vi "tvac_gui.vi"() -> ()   [LabVIEW 2017]
uses:
  <vilib>/httpClient/ClientHandle.ctl
  msg7171_linux.llb/send single message.vi
  <vilib>/httpClient/POSTBuffer.vi
  <vilib>/httpClient/LabVIEWHTTPClient.lvlib
panel:
  out "Index Values":u32[](array[numeric])
  in  "Subtractor":i32=10
  in  "index (col)":i32
  in  "alarm":i32
  in  "NumberTCs":i32=120
  in  "Tab Control":enum32{"Page 1", "Page 2"}(tab)
  in  "Zone 1":T1 {"Ring" items=["Average", "Maximum", "Minimum", ""]}
  in  "Graphing Selection":u16(ring) items=["User Selection", "Graph All Thermocouples", "Clear Graph"]
  in  "Time Scale":u16(ring) items=["Minutes", "Hours", "Seconds"]
  out "Waveform Chart":waveform(dbl)[](graph)
  out "Thermocouples":T2(array[cluster])
  in  "exit":bool
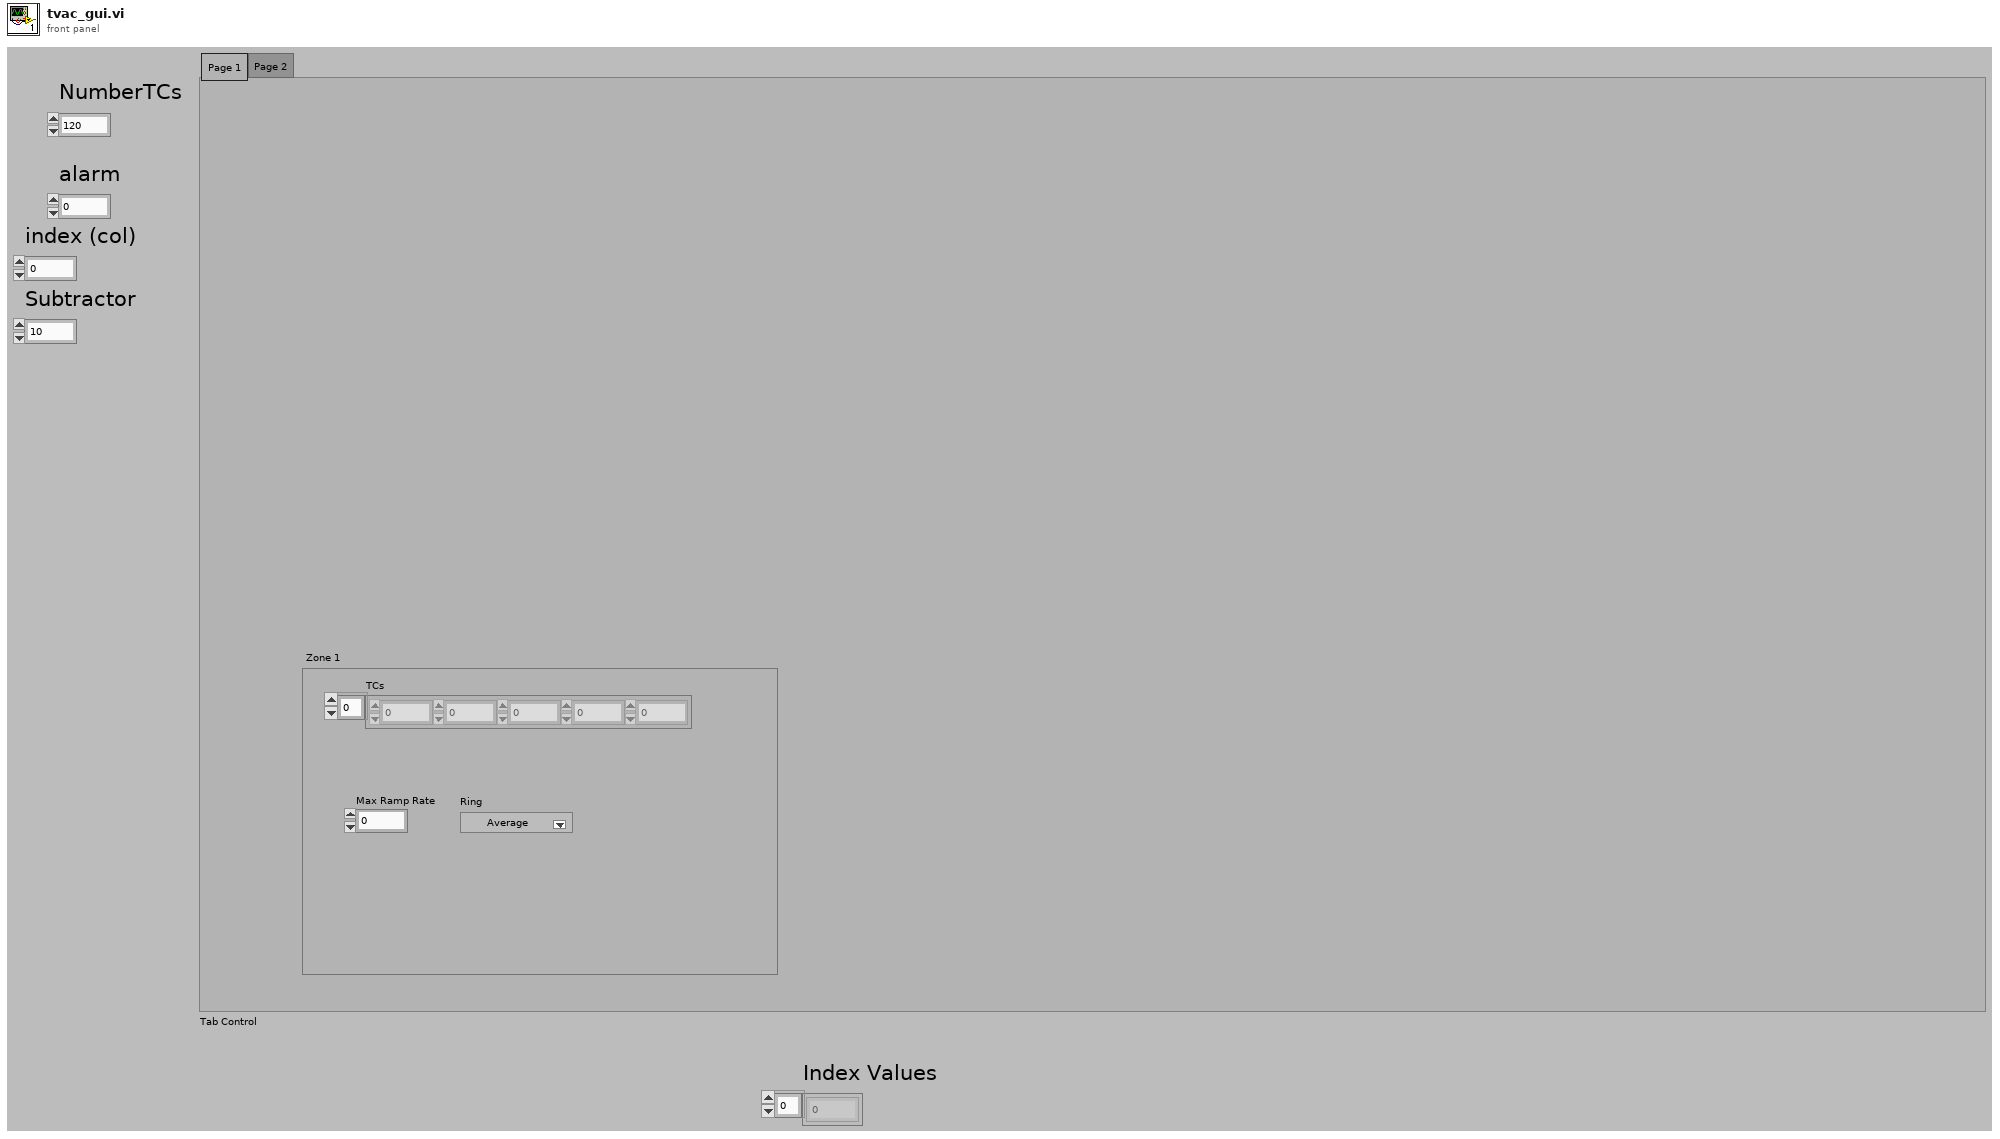
[diagram p1: front panel]
types:
  T1 = cluster{"Ring":u16, "Max Ramp Rate":dbl, "TCs":dbl[]}
  T2 = cluster{"TC Label":string, "Alarm Status":string, "Alarm Color":u32, "Temperature":string, "PlotColor":u32, "Graph On/Off":u32}[][]
  T3 = typedef "LabVIEWHTTPClient.lvlib/ClientHandle.ctl" = refnum<k1>
  T4 = cluster{"go":bool, "Http session":T3, "URL prefex":string}
  T5 = typedef "LVPoint32TypeDef.ctl" = cluster{"Horizontal":i32, "Vertical":i32}
  T6 = typedef "LVPositionTypeDef.ctl" = cluster{"Left":i32, "Top":i32}
  T7 = cluster{"TC Label":string, "Alarm Status":string, "Alarm Color":u32, "Temperature":string, "PlotColor":u32, "Graph On/Off":u32}
  T8 = typedef "LVRangeTypeDef.ctl" = cluster{"Minimum":dbl, "Maximum":dbl, "Increment":dbl, "Minor Increment":dbl, "Start":dbl}
  T9 = cluster{"time":string, "tcs":cluster{"thermocouple":i32, "time":i32, "temp":i32, "working":bool, "alarm":i32}[]}
  T10 = cluster{"thermocouple":i32, "time":i32, "temp":i32, "working":bool, "alarm":i32}[]
  T11 = cluster{"thermocouple":i32, "time":i32, "temp":i32, "working":bool, "alarm":i32}
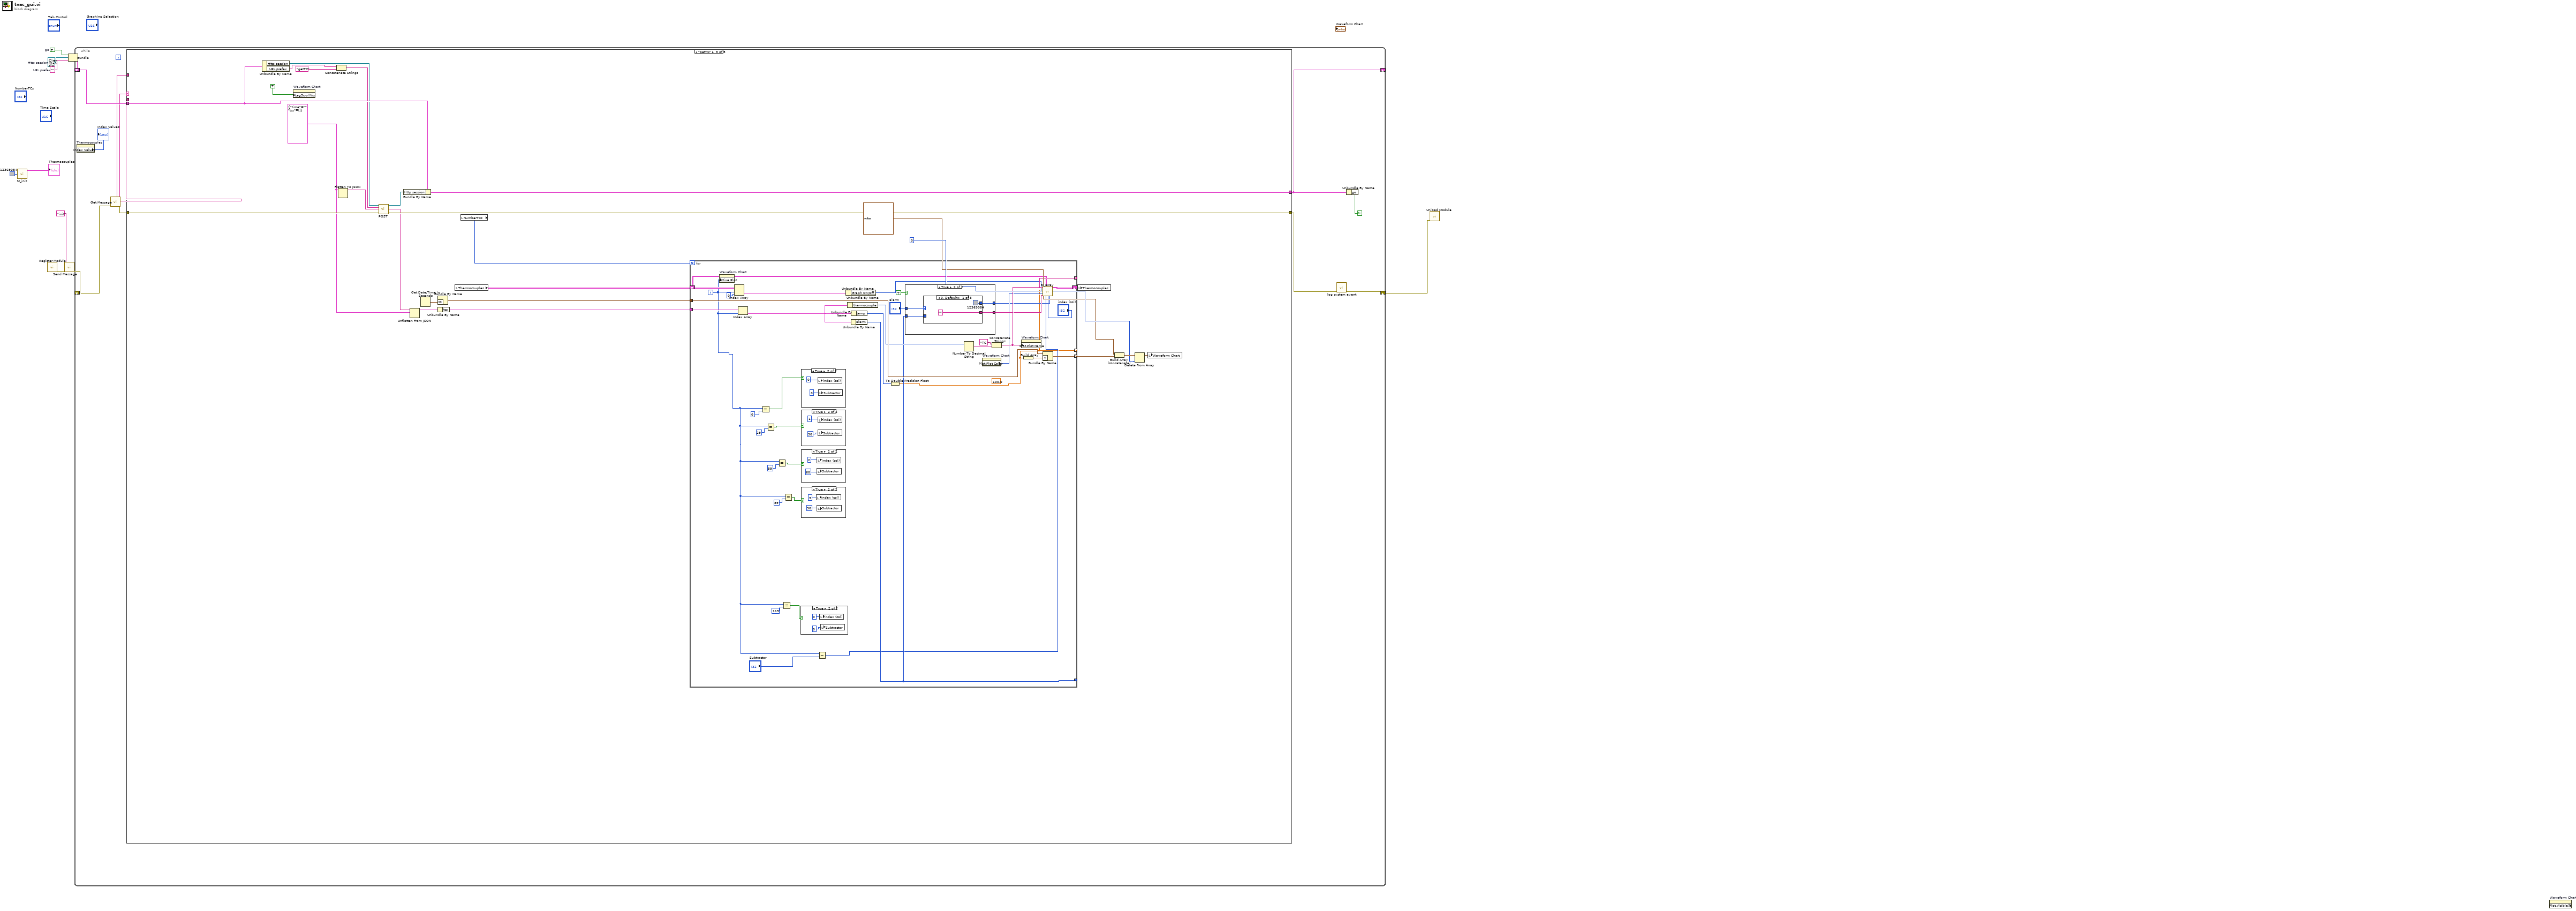
[diagram p0: block diagram]
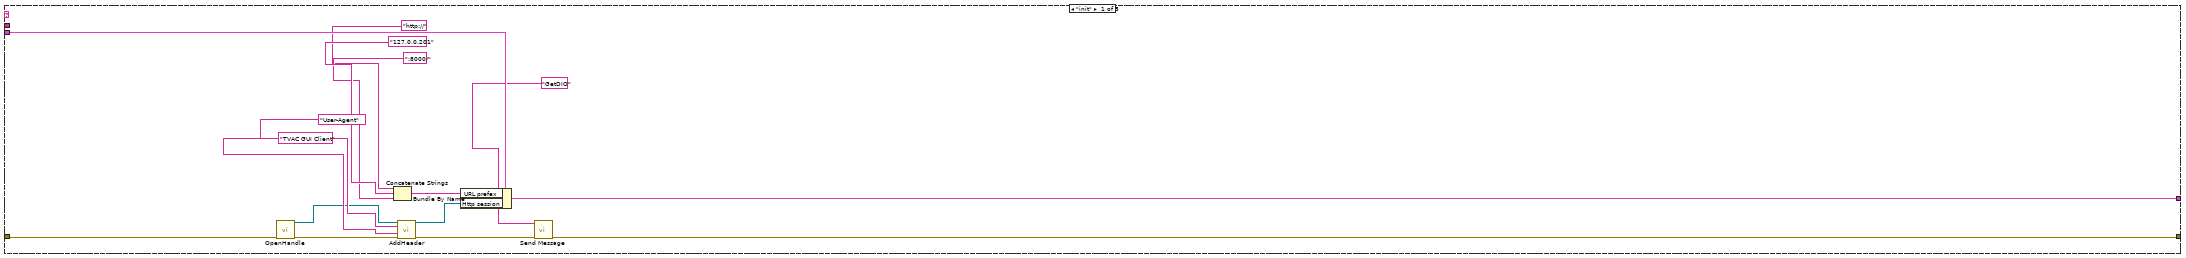
[diagram p2: hidden frame]
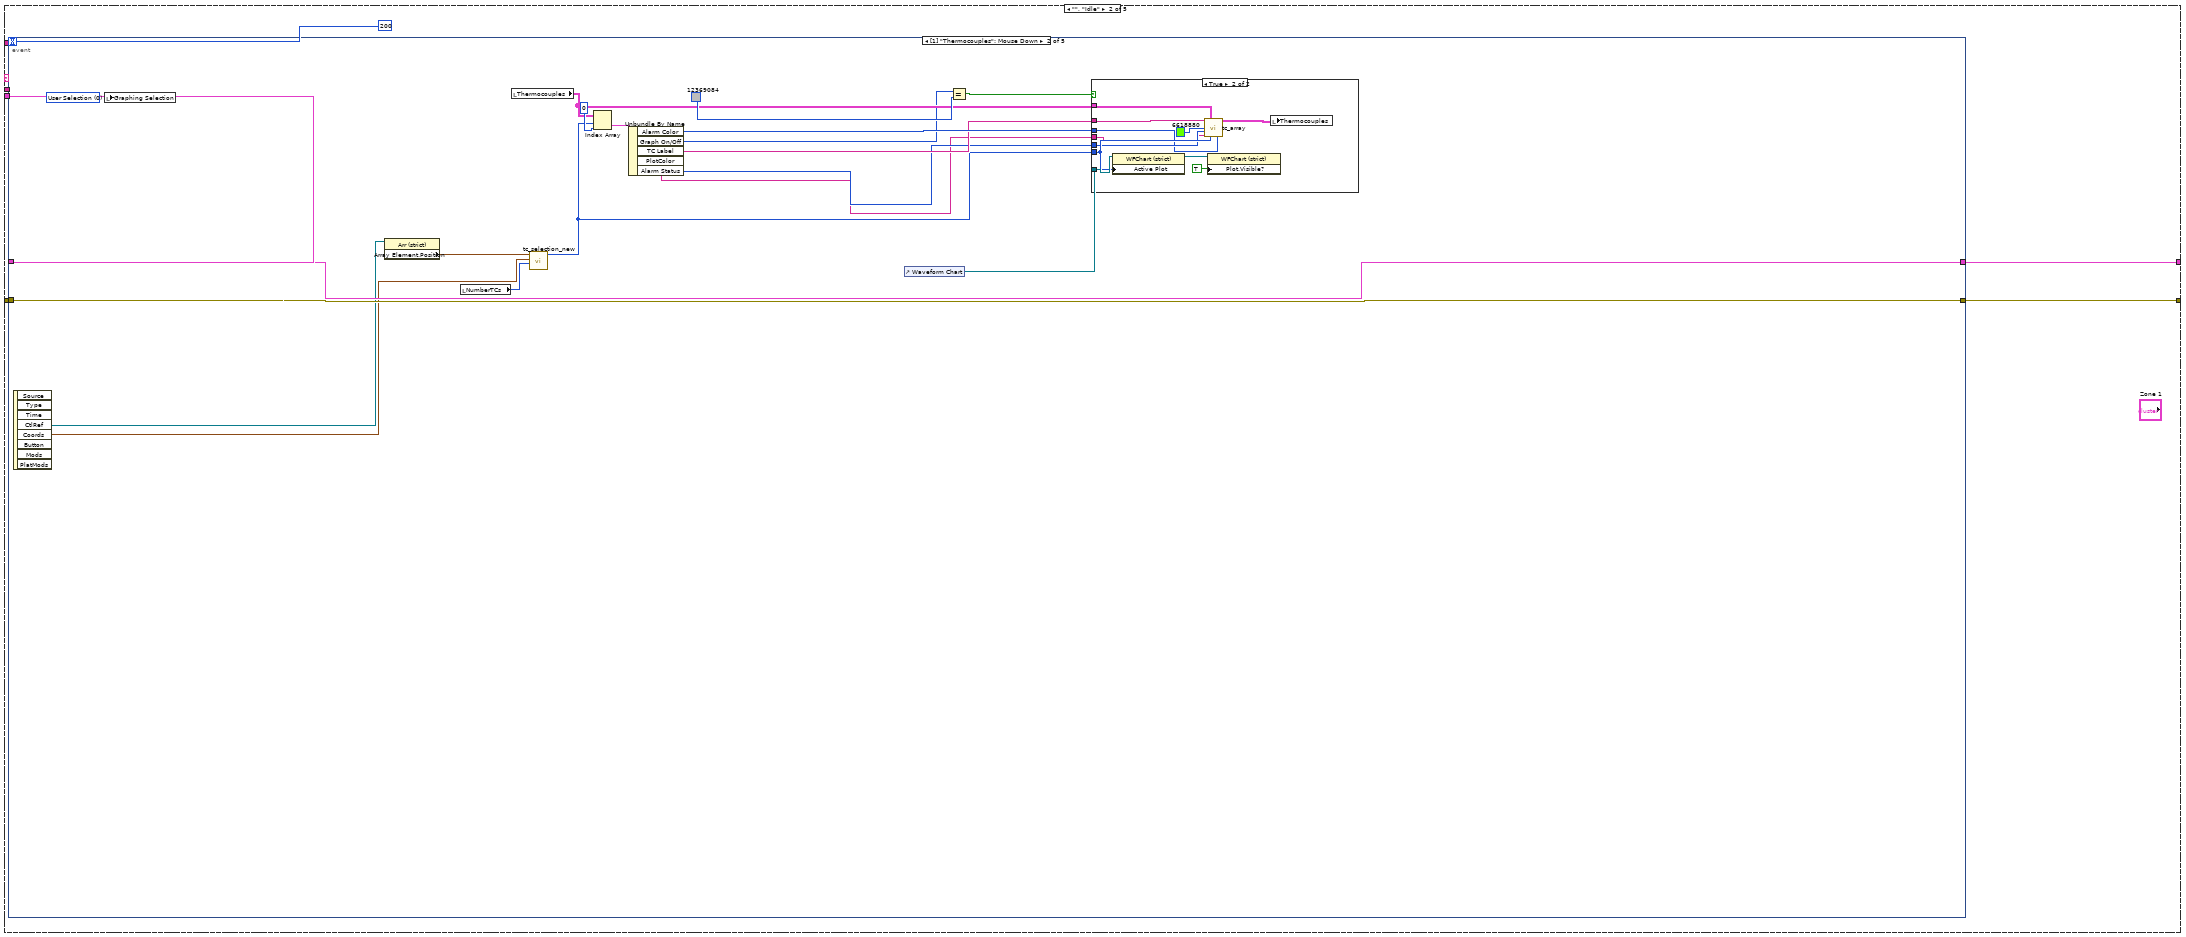
[diagram p3: hidden frame]
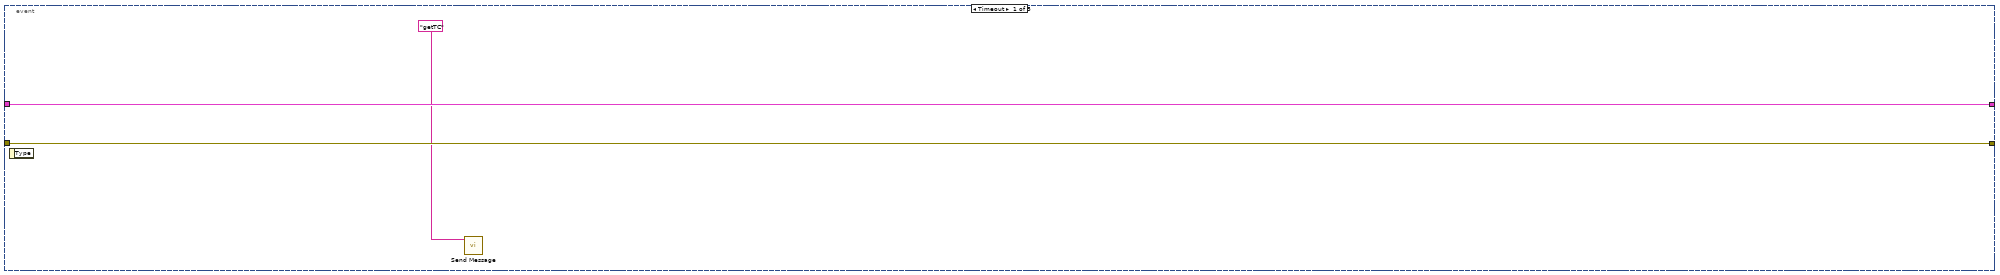
[diagram p4: hidden frame]
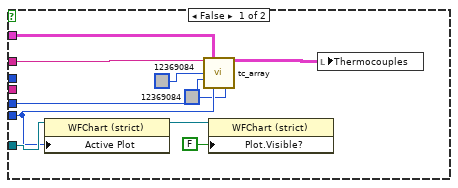
[diagram p5: hidden frame]
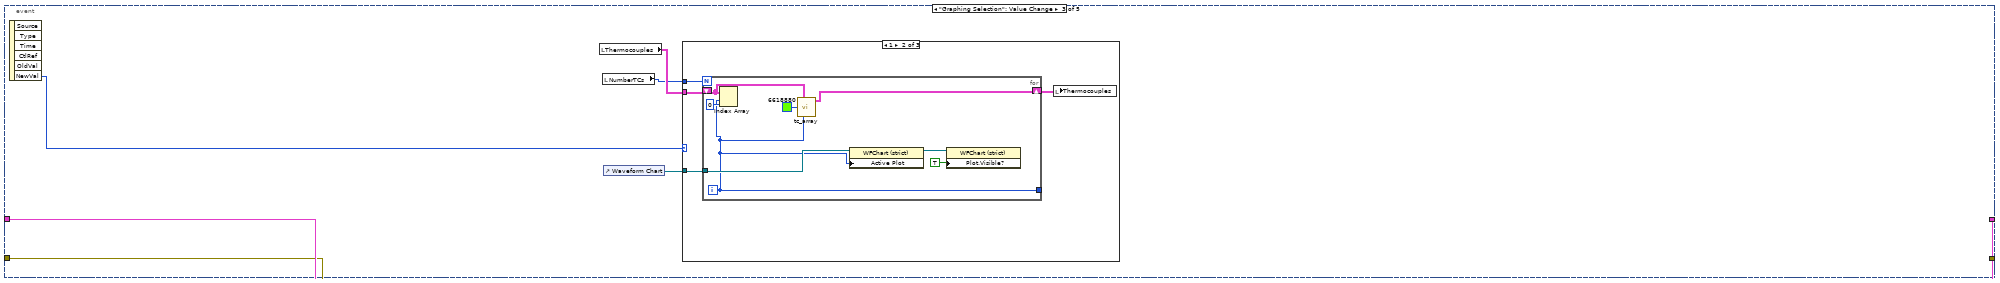
[diagram p6: hidden frame]
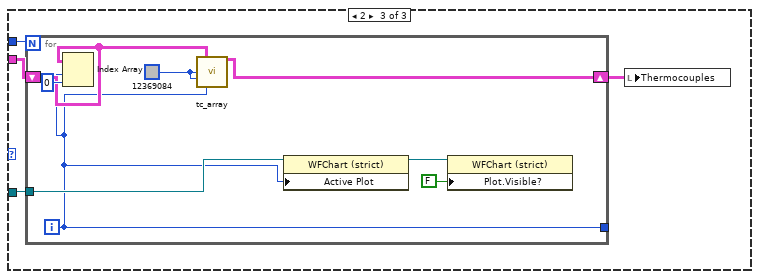
[diagram p8: hidden frame]
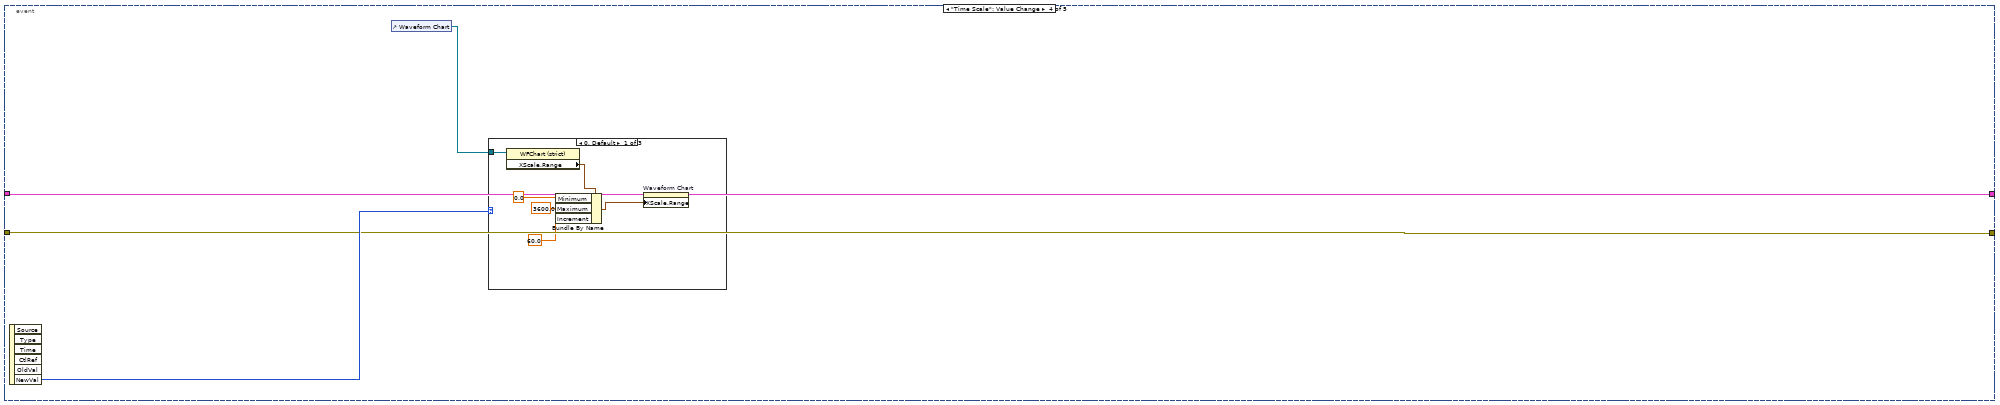
[diagram p9: hidden frame]
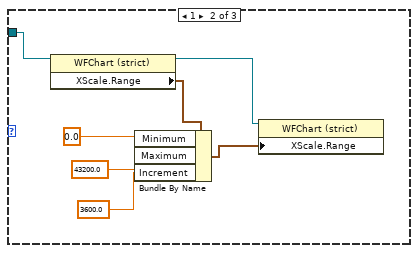
[diagram p10: hidden frame]
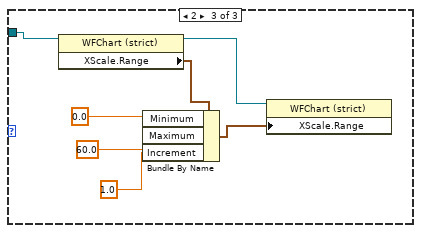
[diagram p11: hidden frame]
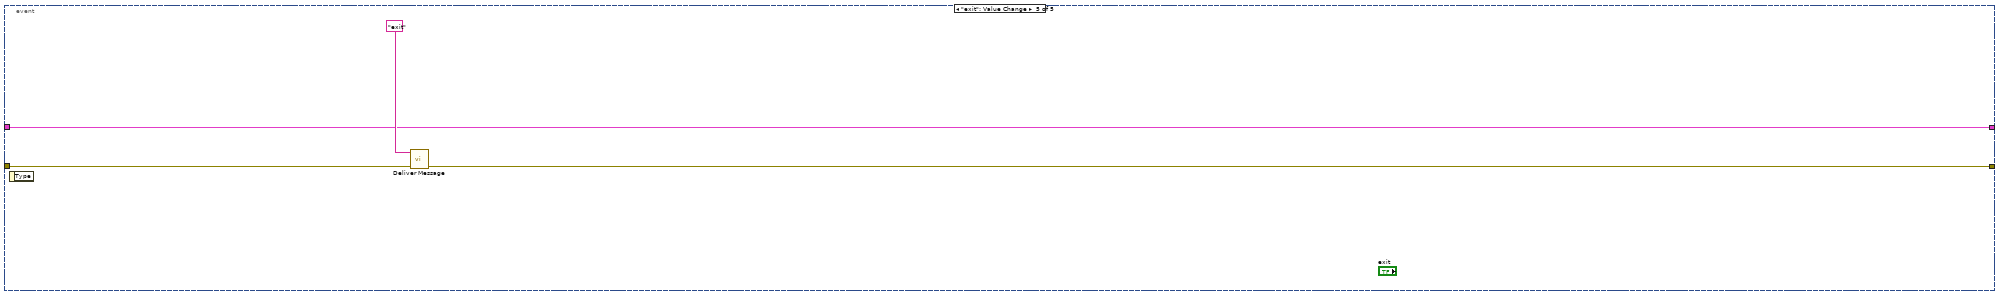
[diagram p12: hidden frame]
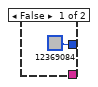
[diagram p18: hidden frame]
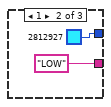
[diagram p19: hidden frame]
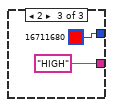
[diagram p20: hidden frame]
diagram:
  w6 = ""  # URL prefex
  w7 = T3 refnum  # Http session
  w8 = TRUE  # go
  n1 = call "tc_init.vi"("Graph ON/OFF"=u32 12369084) -> ("output array"=→"Thermocouples":T2)  [unwired: 14 in]
  n2 = call "Register Module.vi"() -> ("error out"=w4:errorcluster)  [unwired: 10 in, 1 out]
  n3 = call-poly "Send Message.vi"("error in (no error)"=w4, "event"="init") -> ("error out"=w3:errorcluster)  [unwired: 9 in]
  n4 = Bundle("go"=w8, "Http session"=w7, "URL prefex"=w6) -> (w10:T4)  [unwired: 1 in]
  n5 = while {
    shift-left: w10 -> [w18]
    shift-right: [w16] -> _
    shift-right: [w15] -> w9
    shift-left: w3 -> [w21]
    stop <- w12 continue-if-true
    n6 = property on="Thermocouples" class="Arr (strict)"() -> ("Index Values"=→"Index Values":u32[])  [unwired: 2 in, 2 out]
    n7 = call "Get Message.vi"("error in (no error)"=w21) -> ("error out"=w19:errorcluster, "event buffer"=w20:string, "event"=w17:string, "source"=w13:string)  [unwired: 7 in]
    n8 = case shown="\"getTC\"" w17 {
      selector: w17 -> [_ _ _ _ w232]
      tunnel: [w27 w38 w165 w230 w234] -> w16
      tunnel: w18 -> [w36 w37 w163 w225 w234]
      tunnel: w20 -> [_ _ _ _ _]
      tunnel: w19 -> [w31 w39 w167 w228 w233]
      tunnel: [w23 w41 w166 w227 w231] -> w14
      tunnel: w13 -> [_ _ _ _ _]
      frame "init" {
        n9 = call <vilib>:"OpenHandle.vi"("error in (no error)"=w31) -> ("client handle out"=w32:T3, "error out"=w35:errorcluster)  [unwired: 13 in]
        n10 = Concatenate Strings("http://" ("url"), "127.0.0.201" ("Address"), ":8000/" ("url")) -> (w26:string)
        n11 = call <vilib>:"AddHeader.vi"("client handle"=w32, "header"="User-Agent", "value"="TVAC GUI Client", "error in (no error)"=w35) -> ("client handle out"=w25:T3, "error out"=w24:errorcluster)  [unwired: 10 in]
        n12 = Bundle By Name(cluster=w36, "URL prefex"=w26, "Http session"=w25) -> (w27:T4)
        n13 = call-poly "Send Message.vi"("error in (no error)"=w24, "event"="GetDIO") -> ("error out"=w23:errorcluster)  [unwired: 9 in]
      }
      frame "", "Idle" {
        n14 = event shown="[1] \"Thermocouples\": Mouse Down" {
          selector: _ -> [_ _ _ _ _]
          dyn-events: _ -> [_ _ _ _ _]
          timeout: 200 ("milliseconds to wait") -> [_ _ _ _ _]
          tunnel: w39 -> [w43 w63 w89 w116 w142]
          tunnel: [w43 w63 w89 w116 w141] -> w41
          tunnel: [w44 w62 w90 w117 w139] -> w38
          tunnel: w37 -> [w44 w62 w90 w117 w139]
          event Timeout {
            n15 = event-data() -> ()  [unwired: 1 in, 1 out]
            n16 = call-poly "Send Message.vi"("event"="getTC") -> ()  [unwired: 10 in, 1 out]
          }
          event "Thermocouples": Mouse Down {
            w45 = u16 0 items=["User Selection", "Graph All Thermocouples", "Clear Graph"] ("Graphing Selection")
            n17 = event-data() -> ("CtlRef"=w59:refnum<vi>, "Coords"=w60:T5)  [unwired: 1 in, 6 out]
            n18 = local write "Graphing Selection"(w45) -> ()
            n19 = property class="Arr (strict)"(reference=w59) -> ("Array Element.Position"=w61:T6)  [unwired: 1 in, 2 out]
            n20 = local read "NumberTCs"() -> (w51:i32)
            n21 = local read "Thermocouples"() -> (w53:T2)
            n22 = call "tc_selection_new.vi"("Numeric 2"=w51, "Coords"=w60, "Position"=w61) -> ("Numeric"=w47:i32)  [unwired: 8 in]
            n23 = Index Array(array=w53, index (row)=w47, index (col)=0 ("disabled index (col)")) -> (element=w56:T7)
            n24 = Unbundle By Name(w56) -> ("Alarm Color"=w52:u32, "Graph On/Off"=w50:u32, "TC Label"=w49:string, "PlotColor"=w48:u32, "Alarm Status"=w46:string)
            n25 = control-ref of="Waveform Chart"() -> (w54:refnum<vi>)
            n26 = Equal?(x=w50, y=u32 12369084) -> (x = y?=w55:bool)
            n27 = case shown="True" w55 {
              tunnel: w47 -> [w65 w77]
              tunnel: w54 -> [w71 w82]
              tunnel: w53 -> [w67 w79]
              tunnel: w52 -> [_ w74]
              tunnel: w49 -> [w69 w81]
              tunnel: w48 -> [w66 w76]
              tunnel: w46 -> [_ w75]
              frame False {
                n28 = property on="Property Node" class="WFChart (strict)"(reference=w71, "Active Plot"=w65) -> (reference out=w72:refnum<vi>)  [unwired: 1 in, 1 out]
                n29 = call "tc_array.vi"("TC Label"=w69, "output array 2"=w67, "Graph ON/OFF"=u32 12369084, "Plot Color"=w66, "index (row)"=w65, "AlarmColor"=u32 12369084) -> ("output array"=w68:T2)  [unwired: 9 in]
                n30 = property class="WFChart (strict)"(reference=w72, "Plot.Visible?"=FALSE ("Plot.Visible")) -> ()  [unwired: 1 in, 2 out]
                n31 = local write "Thermocouples"(w68) -> ()
              }
              frame True {
                n32 = property class="WFChart (strict)"(reference=w82, "Active Plot"=w77) -> (reference out=w83:refnum<vi>)  [unwired: 1 in, 1 out]
                n33 = call "tc_array.vi"("TC Label"=w81, "output array 2"=w79, "Graph ON/OFF"=u32 6618880, "Plot Color"=w76, "Alarm String"=w75, "index (row)"=w77, "AlarmColor"=w74) -> ("output array"=w78:T2)  [unwired: 8 in]
                n34 = property class="WFChart (strict)"(reference=w83, "Plot.Visible?"=TRUE ("Plot.Visible")) -> ()  [unwired: 1 in, 2 out]
                n35 = local write "Thermocouples"(w78) -> ()
              }
            }
          }
          event "Graphing Selection": Value Change {
            n36 = event-data() -> ("NewVal"=w85:u16)  [unwired: 1 in, 5 out]
            n37 = local read "Thermocouples"() -> (w88:T2)
            n38 = local read "NumberTCs"() -> (w86:i32)
            n39 = control-ref of="Waveform Chart"() -> (w87:refnum<vi>)
            n40 = case shown="1" w85 {
              tunnel: w88 -> [_ w94 w105]
              tunnel: w87 -> [_ w93 w104]
              tunnel: w86 -> [_ w92 w106]
              frame 0, Default {
              }
              frame 1 {
                n41 = for {
                  N: w92 -> [_]
                  tunnel: w93 -> [w99]
                  tunnel: [w98] -> _
                  shift-right: [w96] -> w91
                  shift-left: w94 -> [w97]
                  i -> [w98]
                  n42 = Index Array(array=w97, index (row)=w98, index (col)=0 ("disabled index (col)")) -> ()  [unwired: 1 out]
                  n43 = call "tc_array.vi"("output array 2"=w97, "Graph ON/OFF"=u32 6618880, "index (row)"=w98) -> ("output array"=w96:T2)  [unwired: 12 in]
                  n44 = property class="WFChart (strict)"(reference=w99, "Active Plot"=w98) -> (reference out=w101:refnum<vi>)  [unwired: 1 in, 1 out]
                  n45 = property class="WFChart (strict)"(reference=w101, "Plot.Visible?"=TRUE ("Plot.Visible")) -> ()  [unwired: 1 in, 2 out]
                }
                n46 = local write "Thermocouples"(w91) -> ()
              }
              frame 2 {
                n47 = for {
                  N: w106 -> [_]
                  tunnel: w104 -> [w111]
                  tunnel: [w109] -> _
                  shift-right: [w107] -> w103
                  shift-left: w105 -> [w110]
                  i -> [w109]
                  w108 = u32 12369084
                  n48 = Index Array(array=w110, index (row)=w109, index (col)=0 ("disabled index (col)")) -> ()  [unwired: 1 out]
                  n49 = call "tc_array.vi"("output array 2"=w110, "Graph ON/OFF"=w108, "Plot Color"=w108, "index (row)"=w109) -> ("output array"=w107:T2)  [unwired: 11 in]
                  n50 = property class="WFChart (strict)"(reference=w111, "Active Plot"=w109) -> (reference out=w113:refnum<vi>)  [unwired: 1 in, 1 out]
                  n51 = property class="WFChart (strict)"(reference=w113, "Plot.Visible?"=FALSE ("Plot.Visible")) -> ()  [unwired: 1 in, 2 out]
                }
                n52 = local write "Thermocouples"(w103) -> ()
              }
            }
          }
          event "Time Scale": Value Change {
            n53 = event-data() -> ("NewVal"=w118:u16)  [unwired: 1 in, 5 out]
            n54 = control-ref of="Waveform Chart"() -> (w115:refnum<vi>)
            n55 = case shown="0, Default" w118 {
              tunnel: w115 -> [w122 w126 w133]
              frame 0, Default {
                n56 = property on="Property Node" class="WFChart (strict)"(reference=w122) -> ("XScale.Range"=w124:T8)  [unwired: 1 in, 2 out]
                n57 = Bundle By Name(cluster=w124, "Minimum"=0.0, "Maximum"=3600.0, "Increment"=60.0) -> (w123:T8)
                n58 = property on="Waveform Chart" class="WFChart (strict)"("XScale.Range"=w123) -> ()  [unwired: 2 in, 2 out]
              }
              frame 1 {
                n59 = property on="Property Node" class="WFChart (strict)"(reference=w126) -> (reference out=w125:refnum<vi>, "XScale.Range"=w131:T8)  [unwired: 1 in, 1 out]
                n60 = Bundle By Name(cluster=w131, "Minimum"=0.0, "Maximum"=43200.0, "Increment"=3600.0) -> (w127:T8)
                n61 = property on="Property Node" class="WFChart (strict)"(reference=w125, "XScale.Range"=w127) -> ()  [unwired: 1 in, 2 out]
              }
              frame 2 {
                n62 = property on="Property Node" class="WFChart (strict)"(reference=w133) -> (reference out=w132:refnum<vi>, "XScale.Range"=w138:T8)  [unwired: 1 in, 1 out]
                n63 = Bundle By Name(cluster=w138, "Minimum"=0.0, "Maximum"=60.0, "Increment"=1.0) -> (w134:T8)
                n64 = property on="Property Node" class="WFChart (strict)"(reference=w132, "XScale.Range"=w134) -> ()  [unwired: 1 in, 2 out]
              }
            }
          }
          event "exit": Value Change {
            n65 = event-data() -> ()  [unwired: 1 in, 1 out]
            n66 = call "Deliver Message.vi"("error in (no error)"=w142, "event"="exit") -> ("error out"=w141:errorcluster)  [unwired: 9 in]
          }
        }
      }
      frame "getTC" {
        w143 = T9 {"time"="", "tcs"=[]} ("Cluster")
        n67 = Unbundle By Name(w163) -> ("Http session"=w162:T3, "URL prefex"=w160:string)
        n68 = property on="Waveform Chart" class="WFChart (strict)"("LegScrollVis"=TRUE ("Legend:Scrollbar Visible")) -> ()  [unwired: 2 in, 2 out]
        n69 = Concatenate Strings(w160, "getTC" ("url")) -> (w161:string)
        n70 = Flatten To JSON(anything=w143) -> (JSON string=w158:string)  [unwired: 2 in, 1 out]
        n71 = call-poly <vilib>:"POST.vi"("client handle"=w162, "url"=w161, "buffer"=w158, "error in (no error)"=w167) -> ("client handle out"=w164:T3, "body"=w157:string, "error out"=w166:errorcluster)  [unwired: 8 in, 1 out]
        n72 = Bundle By Name(cluster=w163, "Http session"=w164) -> (w165:T4)
        n73 = Unflatten From JSON(JSON string=w157, type and defaults=w143) -> (value=w156:T9)  [unwired: 5 in, 1 out]
        n74 = Get Date/Time In Seconds() -> (seconds since 1Jan1904=w152:timestamp)
        n75 = Unbundle By Name(w156) -> ("tcs"=w155:T10)
        n76 = Bundle By Name("t0"=w152) -> (w151:waveform(dbl))  [unwired: 1 in]
        n77 = local read "Thermocouples"() -> (w147:T2)
        n78 = local read "NumberTCs"() -> (w144:i32)
        n79 = for {
          N: w144 -> [_]
          tunnel: w155 -> [w203]
          tunnel: w151 -> [w201]
          tunnel: [w202] -> w150 mode=indexing
          tunnel: [w168] -> _ mode=indexing
          tunnel: [w188] -> _ mode=indexing
          tunnel: [w190] -> _ mode=indexing
          shift-right: [w189] -> w148
          shift-left: w147 -> [w187]
          i -> [w169]
          (unwired) 100.0 ("x")
          n80 = property on="Waveform Chart" class="WFChart (strict)"("Active Plot"=w169) -> ()  [unwired: 2 in, 2 out]
          n81 = Index Array(array=w187, index (row)=w169, index (col)=0 ("disabled index (col)")) -> (element=w193:T7)
          n82 = Index Array(array=w203, index=w169) -> (element=w195:T11)
          n83 = Equal?(x=w169, y=0) -> (x = y?=w178:bool)
          n84 = Equal?(x=w169, y=29) -> (x = y?=w176:bool)
          n85 = Equal?(x=w169, y=59) -> (x = y?=w174:bool)
          n86 = Equal?(x=w169, y=119) -> (x = y?=w170:bool)
          n87 = Equal?(x=w169, y=89) -> (x = y?=w172:bool)
          n88 = case shown="True" w170 {
            frame False {
            }
            frame True {
              n89 = local write "index (col)"(0 ("Subtractor")) -> ()
              n90 = local write "Subtractor"(0 ("Subtractor")) -> ()
            }
          }
          n91 = case shown="True" w178 {
            frame False {
            }
            frame True {
              n92 = local write "index (col)"(0) -> ()
              n93 = local write "Subtractor"(0 ("Subtractor")) -> ()
            }
          }
          n94 = case shown="True" w176 {
            frame False {
            }
            frame True {
              n95 = local write "index (col)"(1 ("Subtractor")) -> ()
              n96 = local write "Subtractor"(30 ("Subtractor")) -> ()
            }
          }
          n97 = case shown="True" w174 {
            frame False {
            }
            frame True {
              n98 = local write "index (col)"(2 ("Subtractor")) -> ()
              n99 = local write "Subtractor"(60 ("Subtractor")) -> ()
            }
          }
          n100 = case shown="True" w172 {
            frame False {
            }
            frame True {
              n101 = local write "index (col)"(3 ("Subtractor")) -> ()
              n102 = local write "Subtractor"(90 ("Subtractor")) -> ()
            }
          }
          n103 = Subtract(x=w169, y="Subtractor") -> (x-y=w180:i32)
          n104 = Unbundle By Name(w193) -> ("Graph On/Off"=w184:u32)
          n105 = Unbundle By Name(w195) -> ("thermocouple"=w199:i32)
          n106 = Unbundle By Name(w195) -> ("alarm"=w190:i32)
          n107 = Unbundle By Name(w195) -> ("temp"=w197:i32)
          n108 = To Double Precision Float(number=w197) -> (double precision float=w168:dbl)
          n109 = case shown="True" TRUE {
            tunnel: [_ w218] -> w186
            tunnel: "alarm" -> [_ w217]
            tunnel: w190 -> [_ w216]
            tunnel: [u32 12369084 w215] -> w183
            frame False {
            }
            frame True {
              n110 = case shown="0, Default" w217 {
                tunnel: ["" "LOW" "HIGH"] -> w218
                tunnel: w216 -> [_ _ _]
                tunnel: [u32 12369084 u32 2812927 u32 16711680] -> w215
                frame 0, Default {
                }
                frame 1 {
                }
                frame 2 {
                }
              }
            }
          }
          n111 = Number To Decimal String(number=w199) -> (decimal integer string=w200:string)  [unwired: 1 in]
          n112 = property on="Waveform Chart" class="WFChart (strict)"() -> ("Plot.Plot Color"=w185:u32)  [unwired: 2 in, 2 out]
          n113 = Concatenate Strings("TC " ("string"), w200) -> (w188:string)
          n114 = property on="Waveform Chart" class="WFChart (strict)"("Plot.Plot Name"=w188) -> ()  [unwired: 2 in, 2 out]
          n115 = Build Array(w168) -> (w196:dbl[])
          n116 = call "tc_array.vi"("TC Label"=w188, "output array 2"=w187, "Temperature"=w168, "Graph ON/OFF"=w184, "Plot Color"=w185, "Alarm String"=w186, "index (row)"=w180, "index (col)"="index (col)", "AlarmColor"=w183) -> ("output array"=w189:T2)  [unwired: 6 in]
          n117 = Bundle By Name(cluster=w201, "Y"=w196) -> (w202:waveform(dbl))
        }
        n118 = local write "Thermocouples"(w148) -> ()
        n119 = Build Array (concatenate)(waveform(dbl) {"t0"=timestamp(0 s since 1904-01-01), "dt"=1.0, "Y"=[]} ("element"), w150) -> (w154:waveform(dbl)[])
        n120 = Delete From Array(array=w154, index=0) -> (array with subset deleted=w145:waveform(dbl)[])  [unwired: 1 in, 1 out]
        n121 = local write "Waveform Chart"(w145) -> ()
      }
      frame "exit" {
        n122 = Unbundle By Name(w225) -> ("Http session"=w226:T3)
        n123 = call <vilib>:"CloseHandle.vi"("client handle"=w226, "error in (no error)"=w228) -> ("error out"=w227:errorcluster)  [unwired: 13 in]
        n124 = Bundle By Name(cluster=w225, "go"=FALSE ("Bundle Element")) -> (w230:T4)
      }
      frame Default {
        n125 = call "Unknown Message Dialog.vi"("error in (no error)"=w233, "event name"=w232) -> ("error out"=w231:errorcluster)  [unwired: 9 in]
      }
    }
    n126 = call "log system event.vi"("error in (no error)"=w14) -> ("error out"=w15:errorcluster)  [unwired: 9 in, 1 out]
    n127 = Unbundle By Name(w16) -> ("go"=w12:bool)
  }
  n128 = call "Unload Module.vi"("error in (no error)"=w9) -> ()  [unwired: 10 in, 1 out]
  n129 = property on="Waveform Chart" class="WFChart (strict)" props=["Plot", "Visible?"]() -> ()  [unwired: 2 in, 3 out]
